vi "Post Media Tweet - IMAQ Image.vi"(8 "error in":errorcluster, 9 "PNG String":string, 10 "Tweet":string, 11 "Twitter Handle In":T1={"OAuth Credentials"={"Signature Method"=enum."HMAC-SHA1", "Version"="1.0", "Client"={"Token"="", "Secret"=""}, "Access"={"Token"="", "Secret"=""}}, "since ID"="", "max ID"="", "Screen Name"=""}) -> (0 "error out":errorcluster, 3 "Twitter Handle Out":T1={"OAuth Credentials"={"Signature Method"=enum."HMAC-SHA1", "Version"="1.0", "Client"={"Token"="", "Secret"=""}, "Access"={"Token"="", "Secret"=""}}, "since ID"="", "max ID"="", "Screen Name"=""})   [LabVIEW 2013]
uses:
  <vilib>/LVH/i3 Twitter/Controls/Twitter Handle.ctl
  <vilib>/LVH/i3 OAuth/Controls/OAuth Handle.ctl
  <vilib>/LVH/i3 OAuth/Controls/Signature Method.ctl
  <vilib>/LVH/i3 OAuth/Controls/Credentials.ctl
  <vilib>/LVH/i3 OAuth/Controls/HTTP Method.ctl
  <vilib>/httpClient/MultipartData.ctl
  <vilib>/LVH/i3 OAuth/i3-oauth.lvlib
  <vilib>/httpClient/LabVIEWHTTPClient.lvlib
  <vilib>/LVH/i3 Twitter/i3-twitter.lvlib
panel:
  out "Full URL":string
  out "Header Value":string
  out "body (response)":string
  out "headers (response)":string
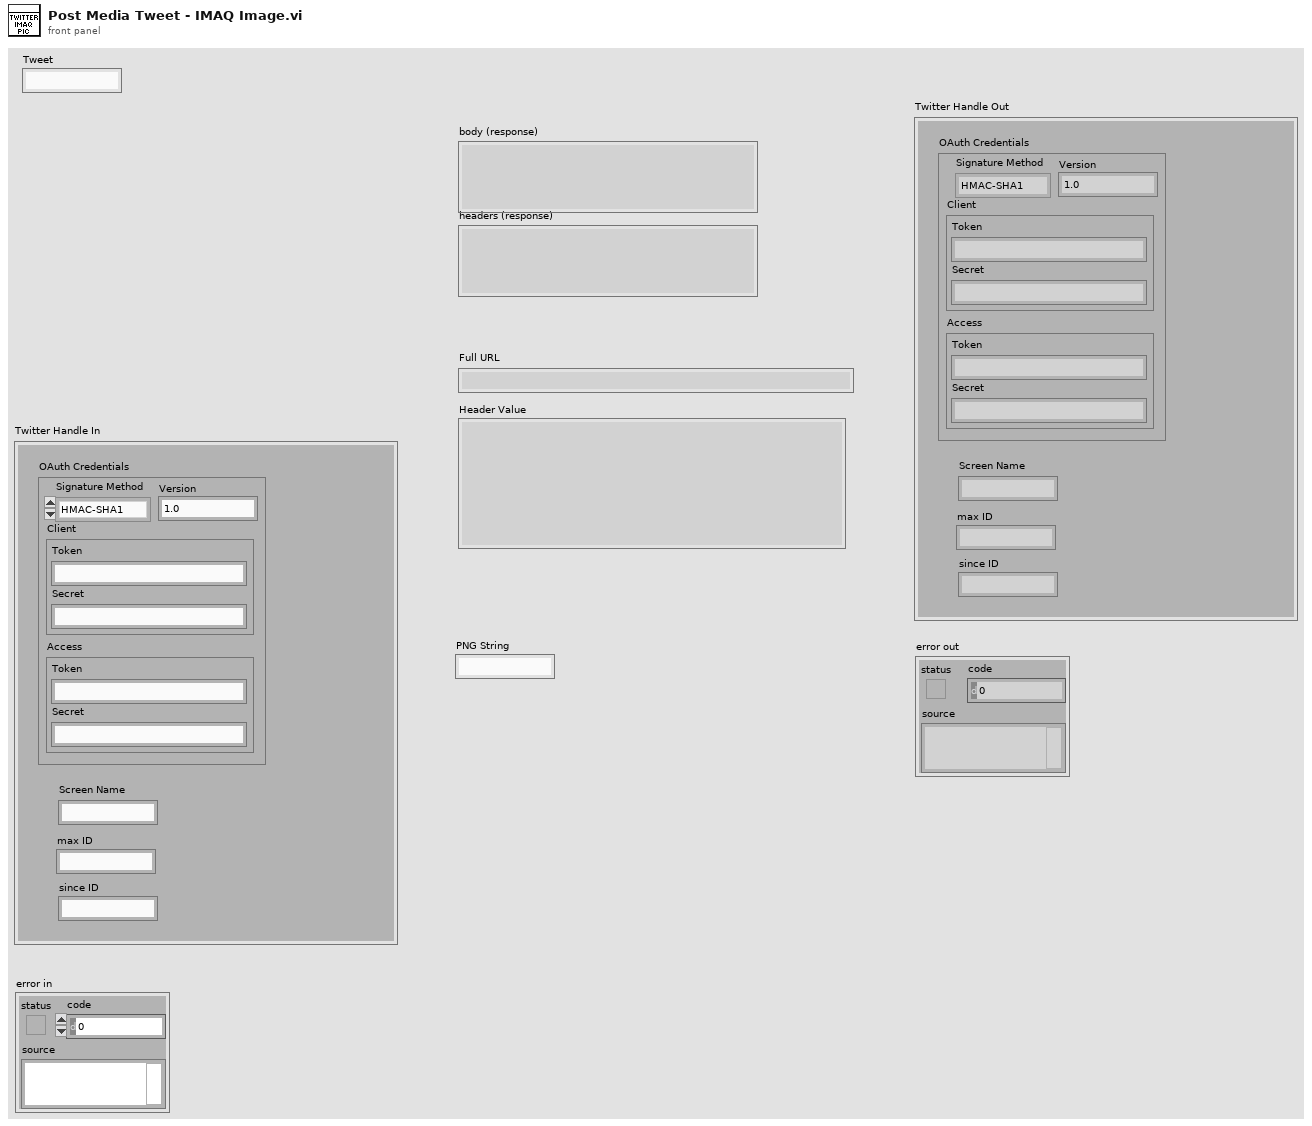
[diagram p1: front panel]
types:
  T1 = typedef "i3-twitter.lvlib/Twitter Handle.ctl" = cluster{"OAuth Credentials":T2, "since ID":string, "max ID":string, "Screen Name":string}
  T2 = typedef "i3-oauth.lvlib/OAuth Handle.ctl" = cluster{"Signature Method":T3, "Version":string, "Client":T4, "Access":T4}
  T3 = typedef "i3-oauth.lvlib/Signature Method.ctl" = enum16{"HMAC-MD5", "HMAC-SHA1", "HMAC-SHA224", "HMAC-SHA256", "HMAC-SHA384", "HMAC-SHA512"}
  T4 = typedef "i3-oauth.lvlib/Credentials.ctl" = cluster{"Token":string, "Secret":string}
  T5 = typedef "LabVIEWHTTPClient.lvlib/MultipartData.ctl" = cluster{"Name":string, "Value":string, "File":path, "Filename":string, "MIME type":string}
  T6 = typedef "i3-oauth.lvlib/HTTP Method.ctl" = enum16{"GET", "POST", "PUT", "DELETE"}
  T7 = typedef "LabVIEWHTTPClient.lvlib/ClientHandle.ctl" = refnum<k1>
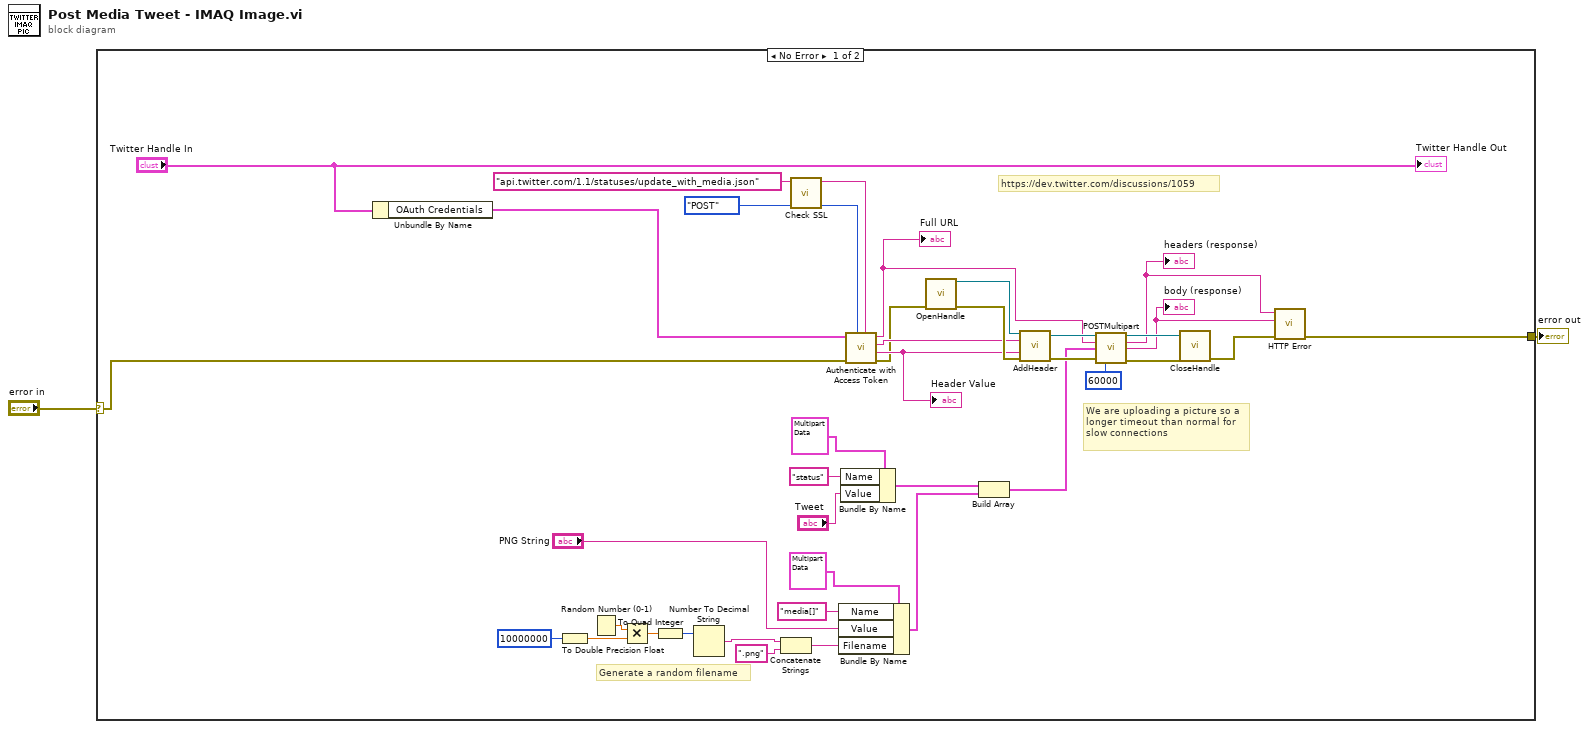
[diagram p0: block diagram]
diagram:
  n1 = case shown="No Error" "error in" {
    selector: "error in" -> [w39 w41]
    tunnel: [w40 w41] -> w2
    frame No Error {
      # "We are uploading a picture so a longer timeout than normal for slow connections"
      # "Generate a random filename"
      # "https://dev.twitter.com/discussions/1059"
      n2 = Unbundle By Name("Twitter Handle In") -> ("OAuth Credentials"=w7:T2)
      n3 = To Double Precision Float(number=10000000) -> (double precision float=w18:dbl)
      n4 = Random Number (0-1)() -> (number: 0 to 1=w20:dbl)
      n5 = Multiply(x=w20, y=w18) -> (x*y=w11:dbl)
      n6 = To Quad Integer(1:w11) -> (0:w10:i64)
      n7 = Number To Decimal String(number=w10) -> (decimal integer string=w14:string)  [unwired: 1 in]
      n8 = Concatenate Strings(w14, ".png" ("string")) -> (w12:string)
      n9 = call <vilib>:"Check SSL.vi"("Input URL"="api.twitter.com/1.1/statuses/update_with_media.json" ("Base URL")) -> ("Output URL"=w5:string)  [unwired: 8 in]
      n10 = Bundle By Name(cluster=T5 {"Name"="", "Value"="", "File"=path "", "Filename"="", "MIME type"="application/octet-stream"} ("Element"), "Name"="media[]", "Value"="PNG String", "Filename"=w12) -> (w23:T5)
      n11 = Bundle By Name(cluster=T5 {"Name"="", "Value"="", "File"=path "", "Filename"="", "MIME type"="application/octet-stream"} ("Element"), "Name"="status", "Value"="Tweet") -> (w27:T5)
      n12 = call <vilib>:"Authenticate with Access Token.vi"("Base URL"=w5, "HTTP Method"=HTTP_Method."POST", "error in (no error)"=w39, "OAuth Handle"=w7) -> ("error out"=w9:errorcluster, "Header Value"=w34:string, "Header Parameter"=w35:string, "Full URL"=w29:string)  [unwired: 3 in, 1 out]
      "Full URL" <- w29
      "Header Value" <- w34
      n13 = call <vilib>:"OpenHandle.vi"("error in (no error)"=w9) -> ("client handle out"=w37:T7, "error out"=w36:errorcluster)  [unwired: 13 in]
      n14 = Build Array(w27, w23) -> (w26:T5[])
      n15 = call <vilib>:"AddHeader.vi"("client handle"=w37, "header"=w35, "value"=w34, "error in (no error)"=w36) -> ("client handle out"=w33:T7, "error out"=w32:errorcluster)  [unwired: 10 in]
      n16 = call <vilib>:"POSTMultipart.vi"("client handle"=w33, "url"=w29, "data"=w26, "error in (no error)"=w32, "timeout (10000)"=60000) -> ("client handle out"=w30:T7, "headers"=w15:string, "body"=w16:string, "error out"=w31:errorcluster)  [unwired: 7 in]
      "body (response)" <- w16
      "headers (response)" <- w15
      n17 = call <vilib>:"CloseHandle.vi"("client handle"=w30, "error in (no error)"=w31) -> ("error out"=w17:errorcluster)  [unwired: 13 in]
      n18 = call <vilib>:"HTTP Error.vi"("error in (no error)"=w17, "Body"=w16, "Header"=w15) -> ("error out"=w40:errorcluster)  [unwired: 6 in, 2 out]
      "Twitter Handle Out" <- "Twitter Handle In"
    }
    frame Error {
    }
  }
  "error out" <- w2
